vi "ObtainBroadcastEvents.vi"(8 "ErrorArray":errorcluster[](array[cluster])) -> (0 "ErrorArray":errorcluster[](array[cluster]), 3 "BusBroadcast":T1)   [LabVIEW 2017, in "Bus_class.lvlib"]
uses:
  Bus_class.lvlib
  Typedefs/clBroadcastEvents.ctl
  Typedefs/clUserEventType.ctl
  <userlib>/NIST/NISTErrorLib/NISTErrorLib.lvlib
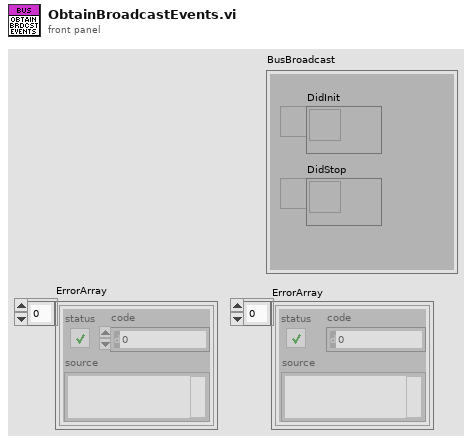
[diagram p1: front panel]
types:
  T1 = typedef "Bus_class.lvlib/clBroadcastEvents.ctl" = cluster{"DidInit":refnum<user-event>, "DidStop":refnum<user-event>}
  T2 = typedef "Bus_class.lvlib/clUserEventType.ctl" = cluster{"BusNumber":i8, "Data":variant}
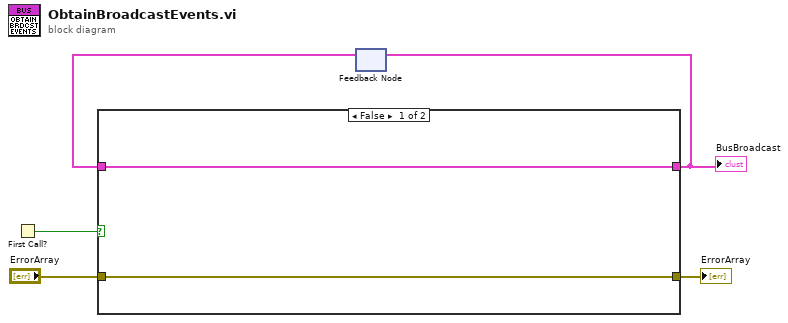
[diagram p0: block diagram]
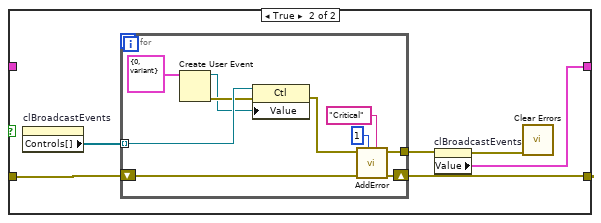
[diagram p2: hidden frame]
diagram:
  n1 = First Call?() -> (First Call?: T/F=w1:bool)
  n2 = feedback #1() -> (w3:T1)  [unwired: 1 in]
  n3 = case shown="False" w1 {
    tunnel: "ErrorArray" -> [w7 w13]
    tunnel: [w7 w12] -> w4
    tunnel: [w6 w9] -> w2
    tunnel: w3 -> [w6 _]
    frame False {
    }
    frame True {
      n4 = property on="clBroadcastEvents" class="Clust (strict)"() -> ("Controls[]"=w11:refnum<vi>[])  [unwired: 2 in, 2 out]
      n5 = for {
        tunnel: w11 -> [w22] mode=indexing
        shift-right: [w16] -> w12
        shift-left: w13 -> [w17]
        tunnel: [w15] -> w8
        n6 = Create User Event(user event datatype=T2 {"BusNumber"=0, "Data"=variant} ("clEventType")) -> (user event=w14:refnum<user-event>, error out=w21:errorcluster)  [unwired: 1 in]
        n7 = property class="Ctl"(reference=w22, error in=w21, "Value"=w14) -> (error out=w18:errorcluster)  [unwired: 1 out]
        n8 = call <userlib>:"AddError.vi"("Severity"="Critical" ("String"), "Priority"=u8 1, "ErrorArray"=w17, "error in (no error)"=w18) -> ("ErrorArray"=w16:errorcluster[], "error out"=w15:errorcluster)  [unwired: 6 in]
      }
      n9 = property on="clBroadcastEvents" class="Clust (strict)"(error in=w8) -> (error out=w10:errorcluster, "Value"=w9:T1)  [unwired: 1 in, 1 out]
      n10 = call <vilib>:"Clear Errors.vi"("error in (no error)"=w10) -> ()  [unwired: 5 in, 2 out]
    }
  }
  "ErrorArray" <- w4
  "BusBroadcast" <- w2
  n11 = feedback-in #1(w2) -> ()
